vi "acquireDoorClosedLimitSignal.vi"(8 "error in (no error)":errorcluster, 10 "Door Context:":T1, 11 "cRIOScanModeTarget in":refnum<class "cRIOScanModeTarget.lvclass">) -> (0 "error out":errorcluster, 2 "doorClosedLimitActiveIsT":bool, 3 "cRIOScanModeTarget out":refnum<class "cRIOScanModeTarget.lvclass">)   [LabVIEW 2012, in "cRIOScanModeTarget.lvclass"]
doc: "Acquires the value of the closed limit signal for the specified door."
uses:
  cRIOScanModeTarget.lvclass
  VentilationDoor/Typedefs/DoorContext.ctl
  VentilationDoor/Typedefs/VCDVentilationDoorTypedefs.lvlib
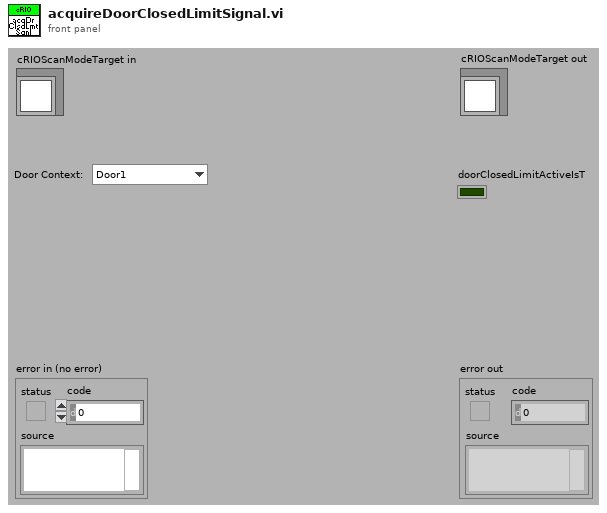
[diagram p1: front panel]
types:
  T1 = typedef "VCDVentilationDoorTypedefs.lvlib/DoorContext.ctl" = enum16{"Door1", "Door2", "Door3", "Door4", "Door5", "Door6", "Door7"}
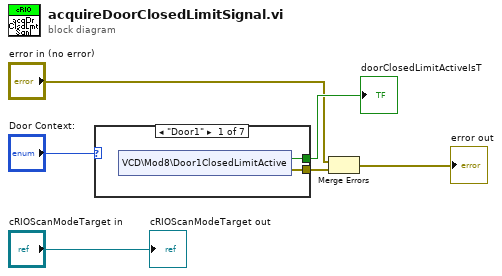
[diagram p0: block diagram]
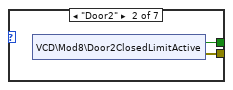
[diagram p2: hidden frame]
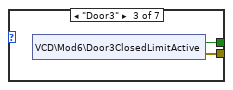
[diagram p3: hidden frame]
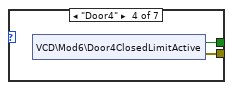
[diagram p4: hidden frame]
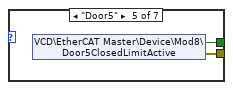
[diagram p5: hidden frame]
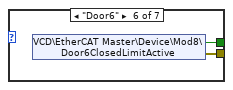
[diagram p6: hidden frame]
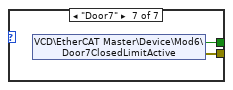
[diagram p7: hidden frame]
diagram:
  n1 = case shown="\"Door1\"" "Door Context:" {
    tunnel: [w8 w10 w12 w14 w16 w18 w20] -> w5
    tunnel: [w7 w9 w11 w13 w15 w17 w19] -> w1
    frame "Door1" {
      n2 = shared-variable "VCD\\Mod8\\Door1ClosedLimitActive"() -> (w8:bool, error out=w7:errorcluster)  [unwired: 1 in]
    }
    frame "Door2" {
      n3 = shared-variable "VCD\\Mod8\\Door2ClosedLimitActive"() -> (w10:bool, error out=w9:errorcluster)  [unwired: 1 in]
    }
    frame "Door3" {
      n4 = shared-variable "VCD\\Mod6\\Door3ClosedLimitActive"() -> (w12:bool, error out=w11:errorcluster)  [unwired: 1 in]
    }
    frame "Door4" {
      n5 = shared-variable "VCD\\Mod6\\Door4ClosedLimitActive"() -> (w14:bool, error out=w13:errorcluster)  [unwired: 1 in]
    }
    frame "Door5" {
      n6 = shared-variable "VCD\\EtherCAT Master\\Device\\Mod8\\Door5ClosedLimitActive"() -> (w16:bool, error out=w15:errorcluster)  [unwired: 1 in]
    }
    frame "Door6" {
      n7 = shared-variable "VCD\\EtherCAT Master\\Device\\Mod8\\Door6ClosedLimitActive"() -> (w18:bool, error out=w17:errorcluster)  [unwired: 1 in]
    }
    frame "Door7" {
      n8 = shared-variable "VCD\\EtherCAT Master\\Device\\Mod6\\Door7ClosedLimitActive"() -> (w20:bool, error out=w19:errorcluster)  [unwired: 1 in]
    }
  }
  "doorClosedLimitActiveIsT" <- w5
  n9 = Merge Errors("error in (no error)", w1) -> (→"error out":errorcluster)
  "cRIOScanModeTarget out" <- "cRIOScanModeTarget in"
